vi "RTM - Apply Tx Configuration.vi"(8 "error in (no error)":errorcluster, 11 "Node Ptr":T1 format="%.0x") -> (0 "error out":errorcluster)   [LabVIEW 2019, in "UDP-Custom-Device System Explorer.lvlib"]
uses:
  UDP-Custom-Device System Explorer.lvlib
  <vilib>/NI VeriStand/Custom Device API/Custom Device Item Ref.ctl
  Shared/Constants.vi
  <vilib>/NI VeriStand/Custom Device API/Set Item Property (Boolean).vi
  <vilib>/NI VeriStand/Custom Device API/Set Item Property (U32).vi
  <vilib>/NI VeriStand/Custom Device API/Custom Device API.lvlib
  Property Accessors/Shared Channel Accessors.lvlib
  Property Accessors/Tx Packet Accessors.lvlib
  Shared/UDP-Custom-Device Shared.lvlib
  Property Accessors/Shared Packet Accessors.lvlib
  <vilib>/NI VeriStand/Custom Device Tools/Custom Device Utility Library/Custom Device Utility Library.lvlib
panel:
  out "Channel Paths":string[](array[string])
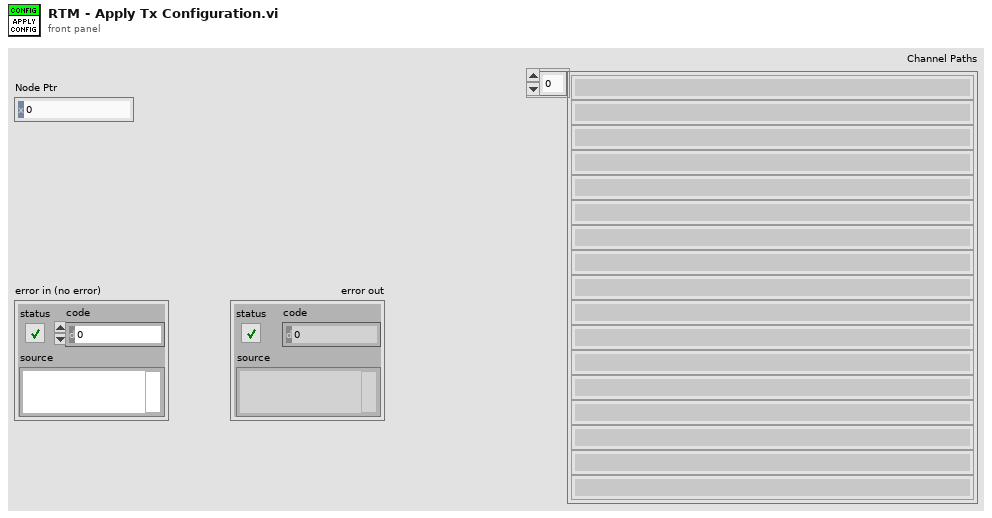
[diagram p1: front panel]
types:
  T1 = typedef "Custom Device API.lvlib/Custom Device Item Ref.ctl" = u64
  T2 = typedef "UDP-Custom-Device Shared.lvlib/Shared - Channel Data Type.ctl" = enum16{"Boolean", "Single", "Double", "I8", "I16", "I32", "I64", "U8", "U16", "U32", "U64"}
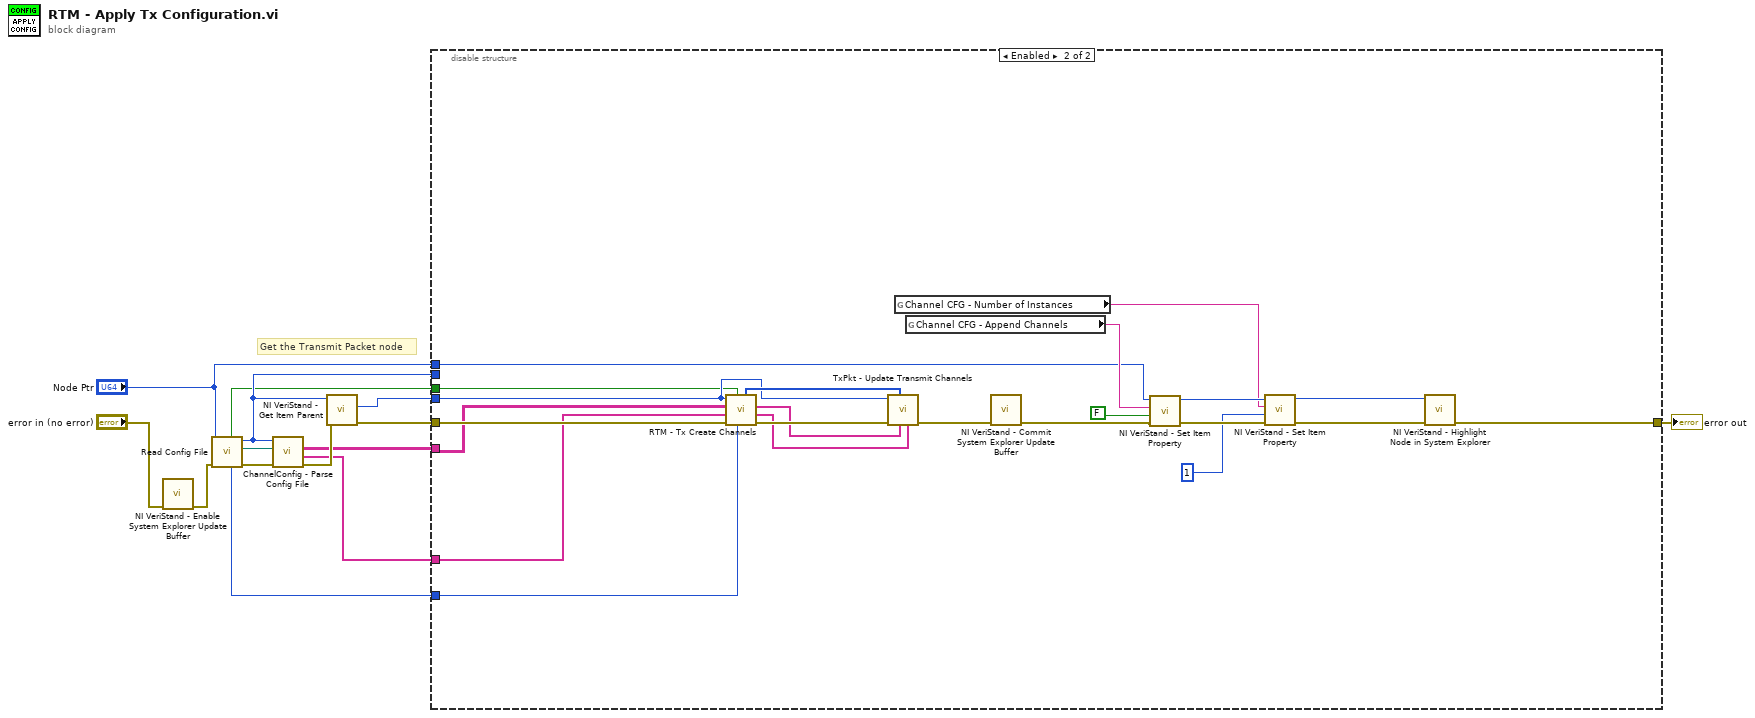
[diagram p0: block diagram]
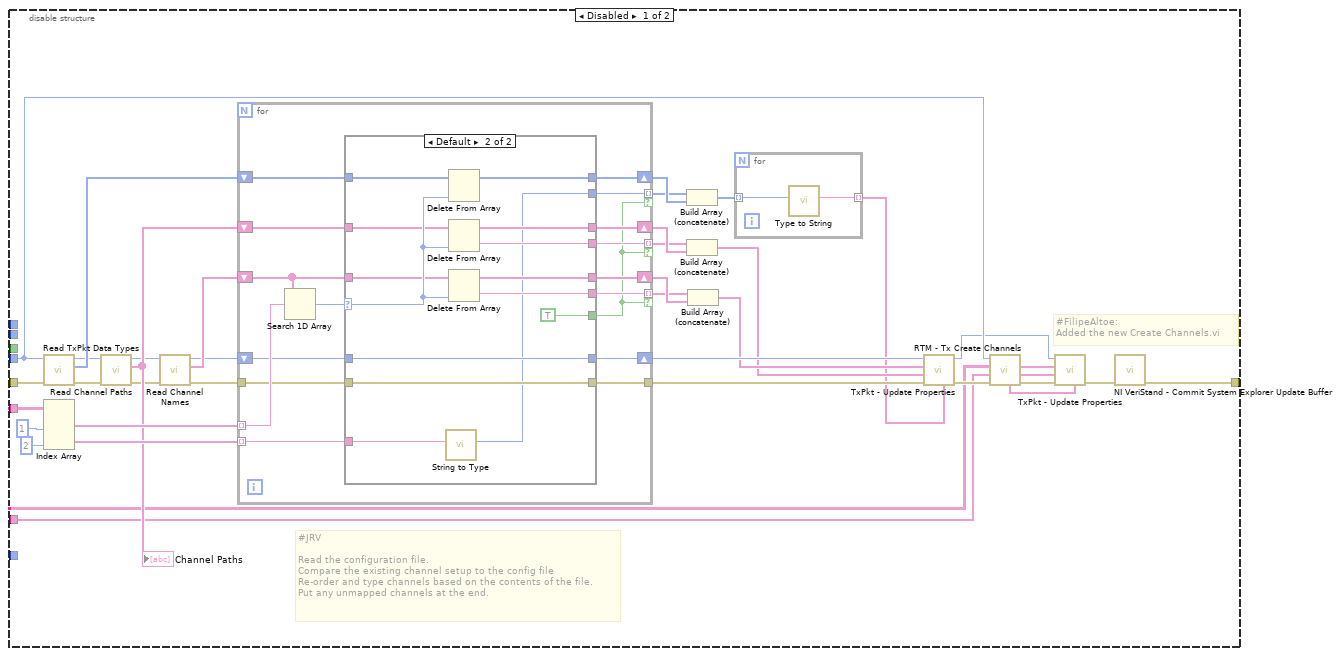
[diagram p2: hidden frame]
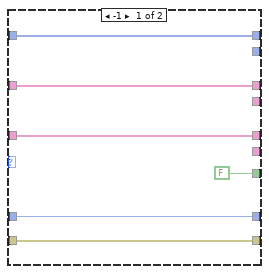
[diagram p3: hidden frame]
diagram:
  # "Get the Transmit Packet node"
  n1 = call <vilib>:"NI VeriStand - Enable System Explorer Update Buffer.vi"("error in (no error)"="error in (no error)") -> ("error out"=w10:errorcluster)  [unwired: 10 in]
  n2 = call "Read Config File.vi"("error in (no error)"=w10, "Node Ptr"="Node Ptr") -> ("error out"=w14:errorcluster, "Config File"=w13:path, "Node Ptr out"=w4:T1, "NumberOfInstances"=w2:u32, "AppendToChannels"=w3:bool)  [unwired: 5 in]
  n3 = call "ChannelConfig - Parse Config File.vi"("error in (no error)"=w14, "Config Path"=w13, "Node Ptr"=w4) -> ("error out"=w12:errorcluster, "Descriptions"=w5:string[], "Channel Configuration"=w6:string[][])  [unwired: 6 in]
  n4 = call <vilib>:"NI VeriStand - Get Item Parent.vi"("error in (no error)"=w12, "Item Ref in"=w4) -> ("error out"=w8:errorcluster, "Parent Ref"=w7:T1)  [unwired: 6 in, 2 out]
  n5 = disable-structure shown="Enabled" {
    disable-tunnel: [w51 w92] -> w9
    disable-tunnel: w8 -> [w46 w112]
    disable-tunnel: w7 -> [w23 w104]
    disable-tunnel: w6 -> [w22 w111]
    disable-tunnel: w5 -> [w21 w110]
    disable-tunnel: w4 -> [_ _]
    disable-tunnel: w3 -> [_ w103]
    disable-tunnel: w2 -> [_ w102]
    disable-tunnel: "Node Ptr" -> [_ w94]
    frame Disabled {
      # "#FilipeAltoe:\nAdded the new Create Channels.vi"
      # "#JRV\n\nRead the configuration file.\nCompare the existing channel setup to the config file\nRe-order and type channels based on the contents of the file.\nPut any unmapped channels at the end."
      n6 = call "Read TxPkt Data Types.vi"("error in (no error)"=w46, "Node Ptr"=w23) -> ("error out"=w31:errorcluster, "Data types"=w47:T2[], "Node Ptr out"=w32:T1)  [unwired: 7 in]
      n7 = Index Array(array=w22, index (col) #1=1 ("disabled index (col)"), index (col) #2=2 ("index (col)")) -> (element #1=w49:string[], element #2=w33:string[])  [unwired: 2 in]
      n8 = call "Read Channel Paths.vi"("error in (no error)"=w31, "Node Ptr"=w32) -> ("error out"=w27:errorcluster, "Channel Paths"=w30:string[], "Node Ptr out"=w28:T1)  [unwired: 7 in]
      "Channel Paths" <- w30
      n9 = call "Read Channel Names.vi"("error in (no error)"=w27, "Node Ptr"=w28) -> ("error out"=w25:errorcluster, "Channel Names"=w29:string[], "Node Ptr out"=w26:T1)  [unwired: 7 in]
      n10 = for {
        tunnel: w49 -> [w70] mode=indexing
        tunnel: w25 -> [w68]
        tunnel: [w69] -> w48
        shift-right: [w62] -> w39
        shift-left: w47 -> [w66]
        shift-right: [w61] -> w41
        shift-left: w30 -> [w65]
        shift-right: [w59] -> w44
        shift-left: w29 -> [w64]
        tunnel: [w63] -> w38 mode=indexing if=w57
        tunnel: [w60] -> w40 mode=indexing if=w57
        tunnel: [w58] -> w42 mode=indexing if=w57
        shift-right: [w56] -> w45
        shift-left: w26 -> [w55]
        tunnel: w33 -> [w54] mode=indexing
        n11 = Search 1D Array(1D array=w64, element=w70) -> (index of element=w67:i32)  [unwired: 1 in]
        n12 = case shown="Default" w67 {
          selector: w67 -> [_ w88]
          tunnel: [w76 w90] -> w69
          tunnel: w68 -> [w76 w90]
          tunnel: w66 -> [w75 w89]
          tunnel: w65 -> [w74 w87]
          tunnel: w64 -> [w73 w86]
          tunnel: [_ w77] -> w63
          tunnel: [w75 w85] -> w62
          tunnel: [w74 w84] -> w61
          tunnel: [_ w83] -> w60
          tunnel: [w73 w82] -> w59
          tunnel: [_ w81] -> w58
          tunnel: [FALSE TRUE] -> w57
          tunnel: [w71 w79] -> w56
          tunnel: w55 -> [w71 w79]
          tunnel: w54 -> [_ w78]
          frame -1 {
          }
          frame Default {
            n13 = call "String to Type.vi"("String Type"=w78) -> ("Data Type"=w77:T2)  [unwired: 10 in]
            n14 = Delete From Array(array=w89, index=w88) -> (array with subset deleted=w85:T2[])  [unwired: 1 in, 1 out]
            n15 = Delete From Array(array=w87, index=w88) -> (deleted portion=w83:string, array with subset deleted=w84:string[])  [unwired: 1 in]
            n16 = Delete From Array(array=w86, index=w88) -> (deleted portion=w81:string, array with subset deleted=w82:string[])  [unwired: 1 in]
          }
        }
      }
      n17 = Build Array (concatenate)(w38, w39) -> (w36:T2[])
      n18 = Build Array (concatenate)(w40, w41) -> (w37:string[])
      n19 = Build Array (concatenate)(w42, w44) -> (w43:string[])
      n20 = for {
        tunnel: w36 -> [w53] mode=indexing
        tunnel: [w52] -> w35 mode=indexing
        n21 = call "Type to String.vi"("Data Type"=w53) -> ("String Type"=w52:string)  [unwired: 10 in]
      }
      n22 = call "TxPkt - Update Properties.vi"("Channel Data Types"=w35, "error in (no error)"=w48, "Channel Paths"=w37, "Channel Names"=w43, "Item Ref in"=w45) -> ("error out"=w24:errorcluster, "Item Ref out"=w18:T1)  [unwired: 5 in]
      n23 = call "RTM - Tx Create Channels.vi"("error in (no error)"=w24, "Descriptions"=w21, "Channel Configuration"=w22, "Node Ptr"=w23) -> ("error out"=w20:errorcluster, "ChannelPaths"=w16:string[], "ChannelNames"=w17:string[], "ChannelDataTypes"=w15:string[])  [unwired: 3 in, 1 out]
      n24 = call "TxPkt - Update Properties.vi"("Channel Data Types"=w15, "error in (no error)"=w20, "Channel Paths"=w16, "Channel Names"=w17, "Item Ref in"=w18) -> ("error out"=w19:errorcluster)  [unwired: 5 in, 1 out]
      n25 = call <vilib>:"NI VeriStand - Commit System Explorer Update Buffer.vi"("error in (no error)"=w19) -> ("error out"=w51:errorcluster)  [unwired: 10 in]
    }
    frame Enabled {
      n26 = call "RTM - Tx Create Channels.vi"("NumberOfInstances"=w102, "AppendToChannels"=w103, "error in (no error)"=w112, "Descriptions"=w110, "Channel Configuration"=w111, "Node Ptr"=w104) -> ("error out"=w108:errorcluster, "ChannelPaths"=w107:string[], "ChannelNames"=w106:string[], "ChannelRefs"=w109:T1[])  [unwired: 1 in, 1 out]
      n27 = call "TxPkt - Update Transmit Channels.vi"("Channel Paths"=w107, "Channel Names"=w106, "Channle Node Refs"=w109, "error in (no error)"=w108, "Node Ptr"=w104) -> ("error out"=w105:errorcluster)  [unwired: 5 in, 1 out]
      n28 = global read "Constants.vi" "Channel CFG - Number of Instances"() -> (w95:string)
      n29 = global read "Constants.vi" "Channel CFG - Append Channels"() -> (w96:string)
      n30 = call <vilib>:"NI VeriStand - Commit System Explorer Update Buffer.vi"("error in (no error)"=w105) -> ("error out"=w100:errorcluster)  [unwired: 10 in]
      n31 = call-poly <vilib>:"NI VeriStand - Set Item Property.vi"("error in (no error)"=w100, "Value"=FALSE, "Property Name"=w96, "Item Ref in"=w94) -> ("error out"=w99:errorcluster, "Item Ref out"=w101:T1)  [unwired: 5 in, 1 out]
      n32 = call-poly <vilib>:"NI VeriStand - Set Item Property.vi"("error in (no error)"=w99, "Value"=u32 1, "Property Name"=w95, "Item Ref in"=w101) -> ("error out"=w93:errorcluster, "Item Ref out"=w91:T1)  [unwired: 5 in, 1 out]
      n33 = call <vilib>:"NI VeriStand - Highlight Node in System Explorer.vi"("error in (no error)"=w93, "Item Ref in"=w91) -> ("error out"=w92:errorcluster)  [unwired: 8 in, 1 out]
    }
  }
  "error out" <- w9
